vi "CanChannelActivate.vi"(3 "error in":errorcluster {"code" format="%.0x"}, 4 "activate":bool, 5 "CAN Channel Handle in":u32 format="%x") -> (0 "error out":errorcluster {"code" format="%.0x"}, 1 "is active":bool, 2 "CAN Channel Handle out":u32)   [LabVIEW 2012]
doc: "Activates or deactivates the CAN message channel."
uses:
  vcilva.dll
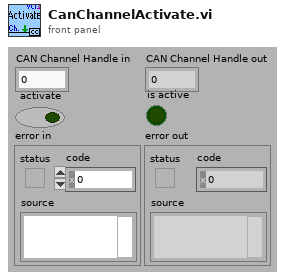
[diagram p1: front panel]
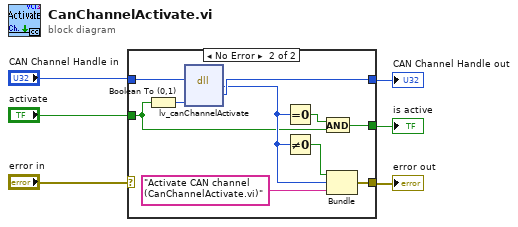
[diagram p0: block diagram]
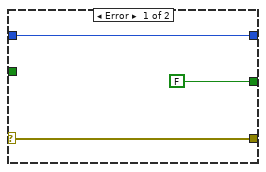
[diagram p2: hidden frame]
diagram:
  n1 = case shown="No Error" "error in" {
    selector: "error in" -> [w8 _]
    tunnel: [w8 w19] -> w3
    tunnel: "CAN Channel Handle in" -> [w9 w15]
    tunnel: [w9 w14] -> w5
    tunnel: [FALSE w10] -> w2
    tunnel: "activate" -> [_ w11]
    frame Error {
    }
    frame No Error {
      n2 = Boolean To (0,1)(Boolean=w11) -> (0, 1=w16:i16)
      n3 = dll-call lib="vcilva.dll" fn="lv_canChannelActivate"("hCanChn"=w15, "fEnable"=w16) -> (w13:i32, "hCanChn"=w14:u32)  [unwired: 4 in, 2 out]
      n4 = Equal To 0?(x=w13) -> (x = 0?=w12:bool)
      n5 = Not Equal To 0?(x=w13) -> (x != 0?=w18:bool)
      n6 = And(x=w12, y=w11) -> (x .and. y?=w10:bool)
      n7 = Bundle(w18, w13, "Activate CAN channel (CanChannelActivate.vi)") -> (w19:errorcluster)  [unwired: 1 in]
    }
  }
  "error out" <- w3
  "CAN Channel Handle out" <- w5
  "is active" <- w2
